vi "PowerSlideOpenTalon.vi"(0 "Controller":T3, 2 "Front Left Channel":T4, 3 "Front Right Channel":T4, 4 "Rear Left Channel":T4, 5 "Rear Right Channel":T4, 6 "Invert Front Left":bool, 7 "PowerSlideReduction":dbl, 8 "Invert Front Right":bool, 9 "PowerSlideTurnThreshold":dbl, 10 "Invert Rear Left":bool, 11 "PowerSlideRatio":bool, 12 "Invert Rear Right":bool) -> (14 "PowerSlideDevRef":T10)   [LabVIEW 2014, in "PowerSlide.lvlib"]
uses:
  PowerSlide.lvlib
  <vilib>/Rock Robotics/SystemInterfaces/Typedef/FPGA_TypedefDigitalModule.ctl
  <vilib>/Rock Robotics/SystemInterfaces/DIO/FPGA_DIOPWMChannel.ctl
  <vilib>/Rock Robotics/WPI/MotorControl/WPI_MotorControlDeviceRef.ctl
  <vilib>/Rock Robotics/WPI/MotorControl/WPI_MotorControlType.ctl
  <vilib>/Rock Robotics/WPI/PWM/WPI_PWMDeadband.ctl
  <vilib>/Rock Robotics/WPI/CAN/Jaguar/SubVIs/WPI_CANJaguar_ControlMode.ctl
  <vilib>/Rock Robotics/WPI/CAN/TalonSRX/WPI_CANTalonSRX_APIControlMode.ctl
  <vilib>/Rock Robotics/WPI/PWM/WPI_PWMTransform_ConPane.ctl
  <vilib>/Rock Robotics/WPI/MotorControl/WPI_MotorControlOpen Talon.vi
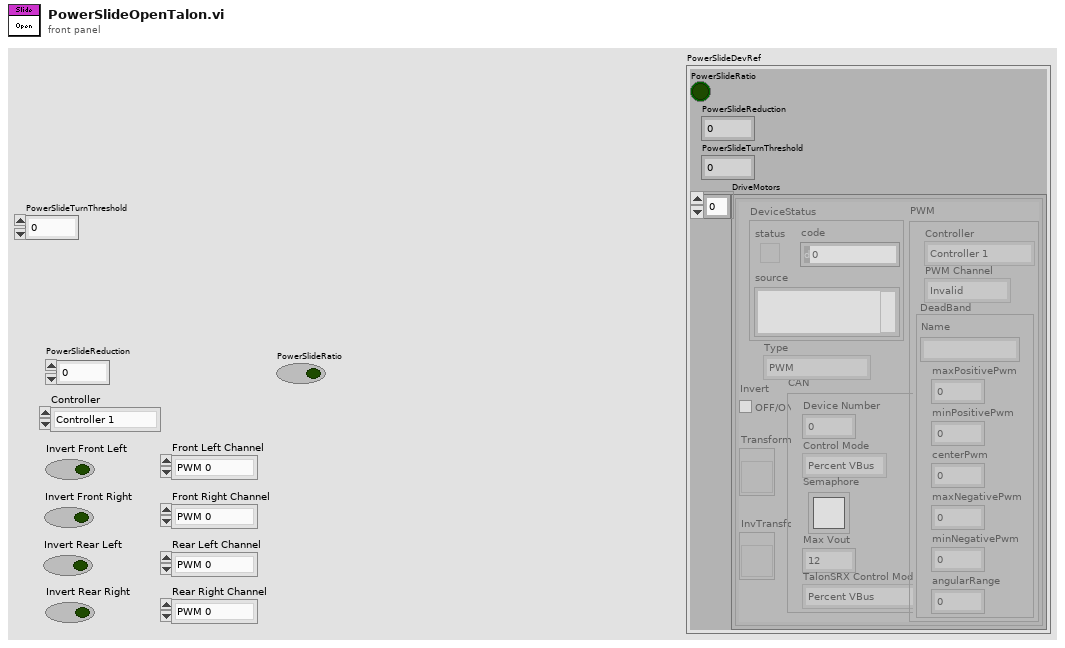
[diagram p1: front panel]
types:
  T1 = typedef "WPI_MotorControlDeviceRef.ctl" = cluster{"DeviceStatus":errorcluster, "Type":T2, "PWM":cluster{"Controller":T3, "PWM Channel":T4, "DeadBand":T5}, "CAN":cluster{"Device Number":u8, "Control Mode":T6, "Semaphore":T7, "Max Vout":dbl, "TalonSRX Control Mode":T8}, "Invert":bool, "TransformRef":T9, "InvTransformRef":T9}
  T2 = typedef "WPI_MotorControlType.ctl" = enum16{"PWM", "CAN", "CANTalonSRX"}
  T3 = typedef "FPGA_TypedefDigitalModule.ctl" = enum16{"Controller 1"}
  T4 = typedef "FPGA_DIOPWMChannel.ctl" = enum8{"PWM 0", "PWM 1", "PWM 2", "PWM 3", "PWM 4", "PWM 5", "PWM 6", "PWM 7", "PWM 8", "PWM 9", "PWM MXP 0", "PWM MXP 1", "PWM MXP 2", "PWM MXP 3", "PWM MXP 4", "PWM MXP 5", "PWM MXP 6", "PWM MXP 7", "PWM MXP 8", "PWM MXP 9", "Invalid"}
  T5 = typedef "WPI_PWMDeadband.ctl" = cluster{"Name":string, "maxPositivePwm":i32, "minPositivePwm":i32, "centerPwm":i32, "maxNegativePwm":i32, "minNegativePwm":i32, "angularRange":u16}
  T6 = typedef "WPI_CANJaguar_ControlMode.ctl" = enum8{"Percent VBus", "Current", "Speed", "Position", "Voltage"}
  T7 = typedef "Semaphore RefNum" = refnum<k1>
  T8 = typedef "WPI_CANTalonSRX_APIControlMode.ctl" = enum8{"Percent VBus", "Speed", "Position", "Slave", "Unchanged / Invalid"}
  T9 = typedef "WPI_PWMTransform_ConPane.ctl" = refnum<vi>
  T10 = cluster{"PowerSlideRatio":bool, "PowerSlideReduction":dbl, "PowerSlideTurnThreshold":dbl, "DriveMotors":T1[]}
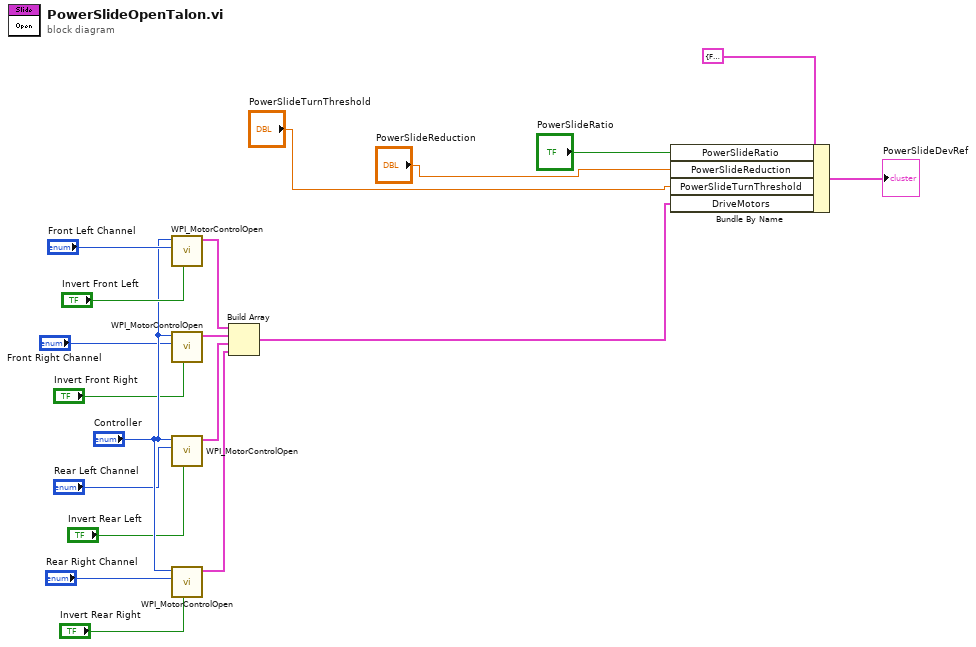
[diagram p0: block diagram]
diagram:
  n1 = call-poly <vilib>:"WPI_MotorControlOpen.vi"("Invert"="Invert Front Left", "PWM Channel"="Front Left Channel", "Controller"="Controller") -> ("MotorControlDeviceRef"=w9:T1)  [unwired: 7 in, 1 out]
  n2 = call-poly <vilib>:"WPI_MotorControlOpen.vi"("Invert"="Invert Front Right", "PWM Channel"="Front Right Channel", "Controller"="Controller") -> ("MotorControlDeviceRef"=w8:T1)  [unwired: 7 in, 1 out]
  n3 = call-poly <vilib>:"WPI_MotorControlOpen.vi"("Invert"="Invert Rear Left", "PWM Channel"="Rear Left Channel", "Controller"="Controller") -> ("MotorControlDeviceRef"=w7:T1)  [unwired: 7 in, 1 out]
  n4 = call-poly <vilib>:"WPI_MotorControlOpen.vi"("Invert"="Invert Rear Right", "PWM Channel"="Rear Right Channel", "Controller"="Controller") -> ("MotorControlDeviceRef"=w6:T1)  [unwired: 7 in, 1 out]
  n5 = Build Array(w9, w8, w7, w6) -> (w2:T1[])
  n6 = Bundle By Name(cluster=T10 {"PowerSlideRatio"=FALSE, "PowerSlideReduction"=0.0, "PowerSlideTurnThreshold"=0.0, "DriveMotors"=[]} ("PowerSlideDevRef"), "PowerSlideRatio"="PowerSlideRatio", "PowerSlideReduction"="PowerSlideReduction", "PowerSlideTurnThreshold"="PowerSlideTurnThreshold", "DriveMotors"=w2) -> (→"PowerSlideDevRef":T10)
